vi "Write.vi"(0 "Logfile Ref In":refnum<file>, 1 "Log":string, 3 "error in (no error)":errorcluster) -> (7 "Logfile Ref Out":refnum<file>, 10 "error out":errorcluster)   [LabVIEW 2016, in "Log4Lv.lvlib"]
doc: "Use this template to build a VI to use as a subVI."
uses:
  Log4Lv.lvlib
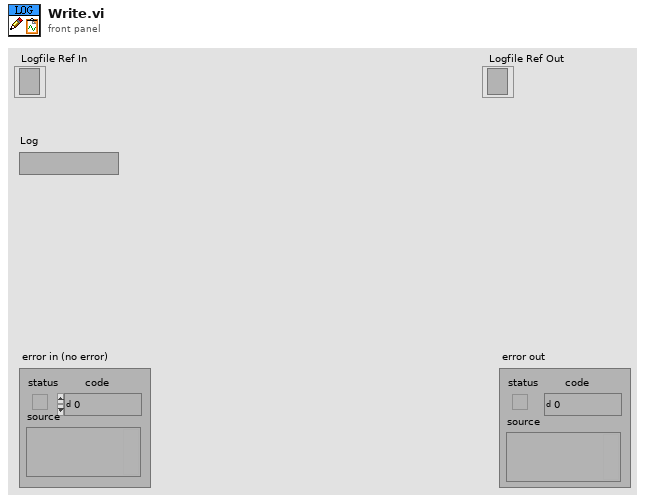
[diagram p1: front panel]
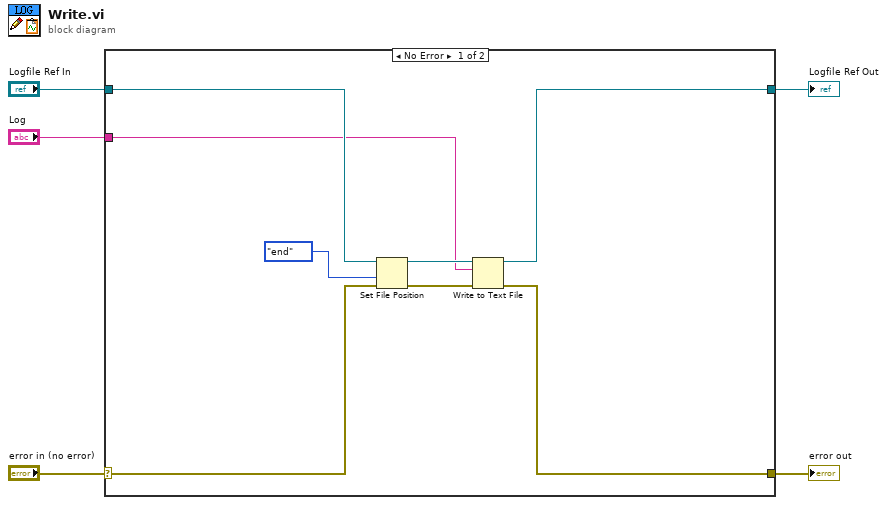
[diagram p0: block diagram]
diagram:
  n1 = case shown="No Error" "error in (no error)" {
    selector: "error in (no error)" -> [w11 w15]
    tunnel: [w7 w15] -> w4
    tunnel: "Logfile Ref In" -> [w13 w14]
    tunnel: "Log" -> [w9 _]
    tunnel: [w6 w14] -> w1
    frame No Error {
      n2 = Set File Position(refnum=w13, from (0:start)=enum16{"start", "end", "current"}."end", error in=w11) -> (refnum out=w10:refnum<file>, error out=w8:errorcluster)  [unwired: 1 in]
      n3 = Write to Text File(file (use dialog)=w10, text=w9, error in=w8) -> (refnum out=w6:refnum<file>, error out=w7:errorcluster)  [unwired: 1 in, 1 out]
    }
    frame Error {
    }
  }
  "error out" <- w4
  "Logfile Ref Out" <- w1
